vi "Remove From VI Info List.vi"(8 "error in":errorcluster, 10 "VI name":string, 11 "state in":T1) -> (0 "error out":errorcluster, 1 "found?":bool, 2 "VI info index":i32, 3 "state out":T1)   [LabVIEW 2010, in "NI_SE_Config Front Panel Layout.lvlib"]
uses:
  NI_SE_Config Front Panel Layout.lvlib
  State.ctl
  VI Info.ctl
  VI Panel Layout/VI Panel Layout.lvclass
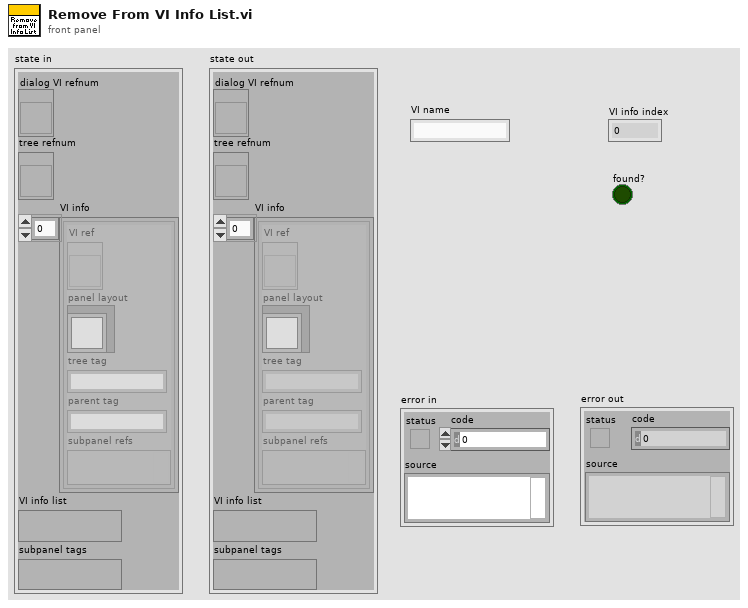
[diagram p1: front panel]
types:
  T1 = typedef "NI_SE_Config Front Panel Layout.lvlib/State.ctl" = cluster{"dialog VI refnum":refnum<vi>, "tree refnum":refnum<vi>, "VI info":T2[], "VI info list":variant, "subpanel tags":variant}
  T2 = typedef "NI_SE_Config Front Panel Layout.lvlib/VI Info.ctl" = cluster{"VI ref":refnum<vi>, "panel layout":refnum<class "VI Panel Layout.lvclass">, "tree tag":string, "parent tag":string, "subpanel refs":variant}
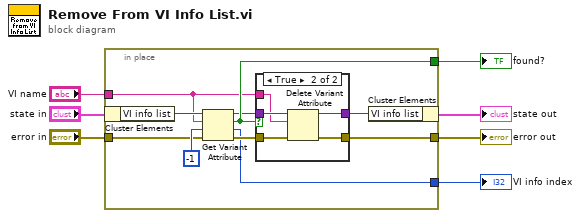
[diagram p0: block diagram]
diagram:
  n1 = in-place {
    in-place-border: "VI name" -> [w12]
    in-place-border: "error in" -> [w15]
    in-place-border: [w14] -> w2
    in-place-border: [w9] -> w4
    in-place-border: [w8] -> w1
    n2 = in-place-cluster #1("state in") -> ("VI info list"=w17:variant)
    n3 = Get Variant Attribute(Variant=w17, name=w12, default value (empty Variant)=-1, error in=w15) -> (duplicate Variant=w13:variant, found=w14:bool, value=w8:i32, error out=w10:errorcluster)
    n4 = case shown="True" w14 {
      tunnel: w13 -> [w19 w24]
      tunnel: w12 -> [_ w23]
      tunnel: [w19 w20] -> w11
      tunnel: w10 -> [w18 w22]
      tunnel: [w18 w21] -> w9
      frame False {
      }
      frame True {
        n5 = Delete Variant Attribute(4:w22, 6:w23, 7:w24) -> (0:w21:errorcluster, 3:w20:variant)  [unwired: 1 out]
      }
    }
    n6 = in-place-cluster #1("VI info list"=w11) -> (→"state out":T1)
  }
  "error out" <- w4
  "VI info index" <- w1
  "found?" <- w2
